vi "Lab6.vi"() -> ()   [LabVIEW 2013]
panel:
  in  "RST":bool
  in  "JC_2":dbl
  out "GANA_J2":bool
  in  "J_2":bool
  out "GANA_J1":bool
  in  "JC_1":dbl
  in  "J_1":bool
  out "C2 4":bool
  out "C2 3":bool
  out "C2 2":bool
  out "C2":bool
  out "C1 4":bool
  out "C1 3":bool
  out "C1 2":bool
  out "C1":bool
  out "Inicio":bool
  in  "stop":bool
  in  "GO":bool
  out "Verde":bool
  out "Amarillo":bool
  out "Rojo":bool
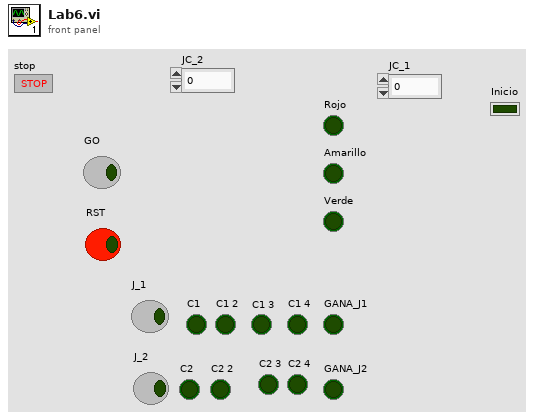
[diagram p1: front panel]
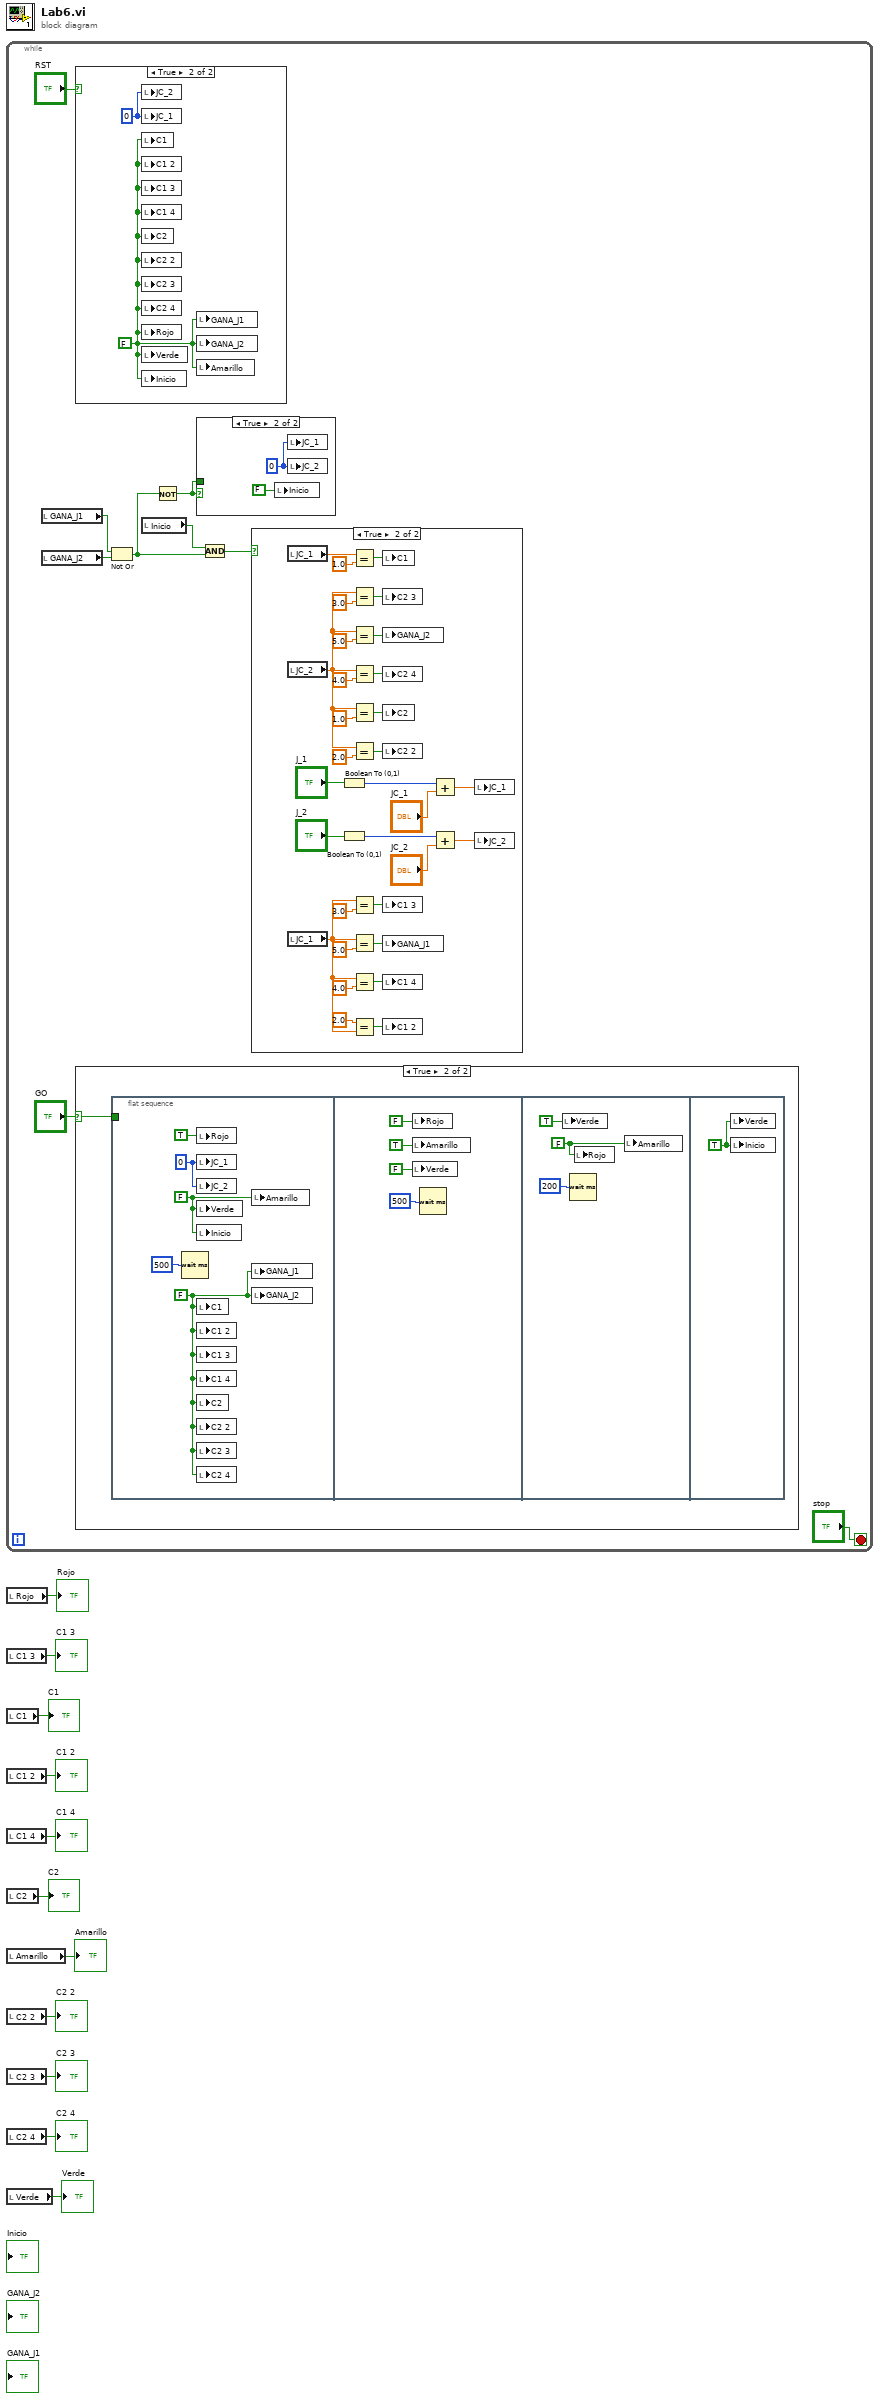
[diagram p0: block diagram]
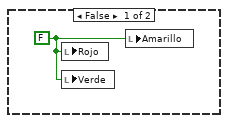
[diagram p5: hidden frame]
diagram:
  n1 = while {
    stop <- "stop" stop-if-true
    n2 = local read "GANA_J1"() -> (w18:bool)
    n3 = local read "GANA_J2"() -> (w17:bool)
    n4 = case shown="True" "RST" {
      frame False {
      }
      frame True {
        w21 = FALSE
        w22 = 0
        n5 = local write "JC_2"(w22) -> ()
        n6 = local write "JC_1"(w22) -> ()
        n7 = local write "C1"(w21) -> ()
        n8 = local write "C1 2"(w21) -> ()
        n9 = local write "C1 3"(w21) -> ()
        n10 = local write "C1 4"(w21) -> ()
        n11 = local write "C2"(w21) -> ()
        n12 = local write "C2 2"(w21) -> ()
        n13 = local write "C2 3"(w21) -> ()
        n14 = local write "C2 4"(w21) -> ()
        n15 = local write "Rojo"(w21) -> ()
        n16 = local write "Verde"(w21) -> ()
        n17 = local write "Inicio"(w21) -> ()
        n18 = local write "GANA_J1"(w21) -> ()
        n19 = local write "GANA_J2"(w21) -> ()
        n20 = local write "Amarillo"(w21) -> ()
      }
    }
    n21 = case shown="True" "GO" {
      selector: "GO" -> [_ w57]
      frame False {
        w56 = FALSE
        n22 = local write "Rojo"(w56) -> ()
        n23 = local write "Verde"(w56) -> ()
        n24 = local write "Amarillo"(w56) -> ()
      }
      frame True {
        n25 = flat-sequence {
          tunnel: w57 -> [_]
          frame #0 {
            w58 = FALSE
            w61 = 0
            w59 = FALSE ("Amarillo")
            n26 = Wait (ms)(milliseconds to wait=u32 500) -> ()  [unwired: 1 out]
            n27 = local write "Rojo"(TRUE ("Rojo")) -> ()
            n28 = local write "JC_1"(w61) -> ()
            n29 = local write "JC_2"(w61) -> ()
            n30 = local write "Verde"(w59) -> ()
            n31 = local write "Inicio"(w59) -> ()
            n32 = local write "C1"(w58) -> ()
            n33 = local write "C1 2"(w58) -> ()
            n34 = local write "C1 3"(w58) -> ()
            n35 = local write "C1 4"(w58) -> ()
            n36 = local write "C2"(w58) -> ()
            n37 = local write "C2 2"(w58) -> ()
            n38 = local write "C2 3"(w58) -> ()
            n39 = local write "C2 4"(w58) -> ()
            n40 = local write "Amarillo"(w59) -> ()
            n41 = local write "GANA_J1"(w58) -> ()
            n42 = local write "GANA_J2"(w58) -> ()
          }
          frame #1 {
            n43 = local write "Rojo"(FALSE ("Rojo")) -> ()
            n44 = local write "Amarillo"(TRUE ("Amarillo")) -> ()
            n45 = local write "Verde"(FALSE ("Verde")) -> ()
            n46 = Wait (ms)(milliseconds to wait=u32 500) -> ()  [unwired: 1 out]
          }
          frame #2 {
            w69 = FALSE ("Rojo")
            n47 = local write "Verde"(TRUE ("Verde")) -> ()
            n48 = Wait (ms)(milliseconds to wait=u32 200) -> ()  [unwired: 1 out]
            n49 = local write "Rojo"(w69) -> ()
            n50 = local write "Amarillo"(w69) -> ()
          }
          frame #3 {
            w70 = TRUE ("Verde")
            n51 = local write "Verde"(w70) -> ()
            n52 = local write "Inicio"(w70) -> ()
          }
        }
      }
    }
    n53 = Not Or(1:w17, 2:w18) -> (0:w13:bool)
    n54 = local read "Inicio"() -> (w16:bool)
    n55 = Not(x=w13) -> (.not. x?=w14:bool)
    n56 = case shown="True" w14 {
      tunnel: w14 -> [_ _]
      frame False {
      }
      frame True {
        w23 = 0
        n57 = local write "Inicio"(FALSE ("Inicio")) -> ()
        n58 = local write "JC_1"(w23) -> ()
        n59 = local write "JC_2"(w23) -> ()
      }
    }
    n60 = And(x=w16, y=w13) -> (x .and. y?=w15:bool)
    n61 = case shown="True" w15 {
      frame False {
      }
      frame True {
        n62 = local read "JC_1"() -> (w51:dbl)
        n63 = local read "JC_2"() -> (w36:dbl)
        n64 = local read "JC_1"() -> (w42:dbl)
        n65 = Boolean To (0,1)(Boolean="J_1") -> (0, 1=w54:i16)
        n66 = Boolean To (0,1)(Boolean="J_2") -> (0, 1=w39:i16)
        n67 = Equal?(x=w51, y=1.0) -> (x = y?=w25:bool)
        n68 = Equal?(x=w36, y=3.0) -> (x = y?=w28:bool)
        n69 = Equal?(x=w36, y=5.0) -> (x = y?=w30:bool)
        n70 = Equal?(x=w36, y=4.0) -> (x = y?=w29:bool)
        n71 = Equal?(x=w36, y=1.0) -> (x = y?=w26:bool)
        n72 = Equal?(x=w36, y=2.0) -> (x = y?=w27:bool)
        n73 = Equal?(x=w42, y=3.0) -> (x = y?=w48:bool)
        n74 = Equal?(x=w42, y=5.0) -> (x = y?=w46:bool)
        n75 = Equal?(x=w42, y=4.0) -> (x = y?=w47:bool)
        n76 = Equal?(x=2.0, y=w42) -> (x = y?=w49:bool)
        n77 = local write "C1"(w25) -> ()
        n78 = local write "C2 3"(w28) -> ()
        n79 = local write "GANA_J2"(w30) -> ()
        n80 = local write "C2 4"(w29) -> ()
        n81 = local write "C2"(w26) -> ()
        n82 = local write "C2 2"(w27) -> ()
        n83 = local write "C1 3"(w48) -> ()
        n84 = local write "GANA_J1"(w46) -> ()
        n85 = local write "C1 4"(w47) -> ()
        n86 = local write "C1 2"(w49) -> ()
        n87 = Add(x=w54, y="JC_1") -> (x+y=w52:dbl)
        n88 = Add(x=w39, y="JC_2") -> (x+y=w37:dbl)
        n89 = local write "JC_1"(w52) -> ()
        n90 = local write "JC_2"(w37) -> ()
      }
    }
  }
  n91 = local read "Rojo"() -> (→"Rojo":bool)
  n92 = local read "C1 3"() -> (→"C1 3":bool)
  n93 = local read "C1"() -> (→"C1":bool)
  n94 = local read "C1 2"() -> (→"C1 2":bool)
  n95 = local read "C1 4"() -> (→"C1 4":bool)
  n96 = local read "C2"() -> (→"C2":bool)
  n97 = local read "Amarillo"() -> (→"Amarillo":bool)
  n98 = local read "C2 2"() -> (→"C2 2":bool)
  n99 = local read "C2 3"() -> (→"C2 3":bool)
  n100 = local read "C2 4"() -> (→"C2 4":bool)
  n101 = local read "Verde"() -> (→"Verde":bool)
